vi "Write Error to FIle.vi"(8 "error in":errorcluster, 11 "error Cluster":T1) -> (0 "error out":errorcluster)   [LabVIEW 2018, in "Error Handler.lvlib"]
doc: "Write the error to a suitable file location"
uses:
  Error Handler.lvlib
  Public Controls/error cluster.ctl
  <vilib>/Utility/file.llb/Write Delimited Spreadsheet (string).vi
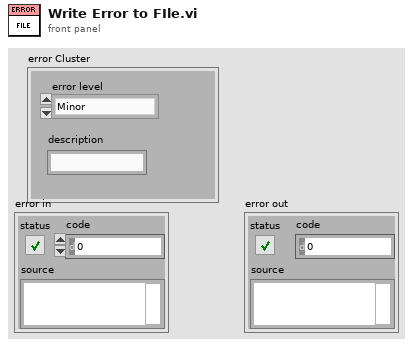
[diagram p1: front panel]
types:
  T1 = typedef "Error Handler.lvlib/error cluster.ctl" = cluster{"error level":enum16{"Minor", "Wash Cycloe", "System Error"}, "description":string}
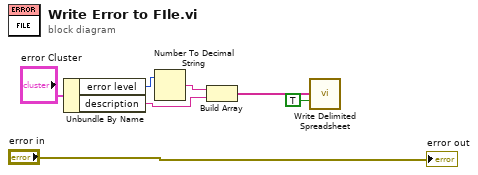
[diagram p0: block diagram]
diagram:
  n1 = Unbundle By Name("error Cluster") -> ("error level"=w5:enum16{"Minor", "Wash Cycloe", "System Error"}, "description"=w3:string)
  n2 = Number To Decimal String(number=w5) -> (decimal integer string=w4:string)  [unwired: 1 in]
  n3 = Build Array(w4, w3) -> (w2:string[])
  n4 = call-poly <vilib>:"Write Delimited Spreadsheet.vi"("1D data"=w2, "append to file? (new file:F)"=TRUE) -> ()  [unwired: 12 in, 2 out]
  "error out" <- "error in"
